vi "Destroy User Events.vi"(11 "UI Template in":refnum<class "Stage Controller.lvclass">) -> (3 "UI Template out":refnum<class "Stage Controller.lvclass">)   [LabVIEW 2020, in "Stage.lvlib" / "Stage Controller.lvlib" / "Stage Controller.lvclass"]
uses:
  Stage Controller.lvclass
  Stage Controller.lvclass/Stage Controller.ctl
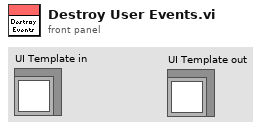
[diagram p1: front panel]
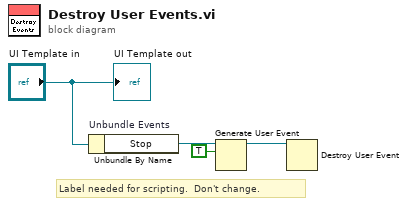
[diagram p0: block diagram]
diagram:
  # "Label needed for scripting.  Don't change."
  n1 = Unbundle By Name "Unbundle Events"("UI Template in") -> ("Stop"=w2:refnum<user-event>)
  n2 = Generate User Event(user event=w2, event data cluster=TRUE ("event data")) -> (user event out=w3:refnum<user-event>)  [unwired: 2 in, 1 out]
  n3 = Destroy User Event(user event=w3) -> ()  [unwired: 1 in, 1 out]
  "UI Template out" <- "UI Template in"
